vi "controls_disable_status.vi"(8 "Controls[]":refnum<vi>[][](array[refnum]), 11 "motions":T1[](array[typedef])) -> ()   [LabVIEW 2016, in "MotionControl.lvlib"]
uses:
  <userlib>/MotionControl/MotionControl.lvlib
  <userlib>/MotionControl/MotorSystem/MotionCluster.ctl
  <userlib>/MotionControl/OneMotion/OneMotion.lvclass
  <userlib>/MotionControl/MotorSystem/MotorSystem.lvclass
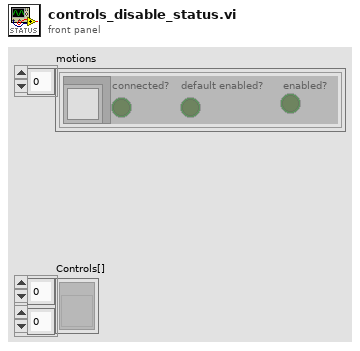
[diagram p1: front panel]
types:
  T1 = typedef "MotionControl.lvlib/MotorSystem.lvclass/MotionCluster.ctl" = cluster{"OneMotion.lvclass":refnum<class "OneMotion.lvclass">, "connected?":bool, "default enabled?":bool, "enabled?":bool}
  T2 = enum8{"Enabled", "Disabled", "Disabled and Grayed Out"}
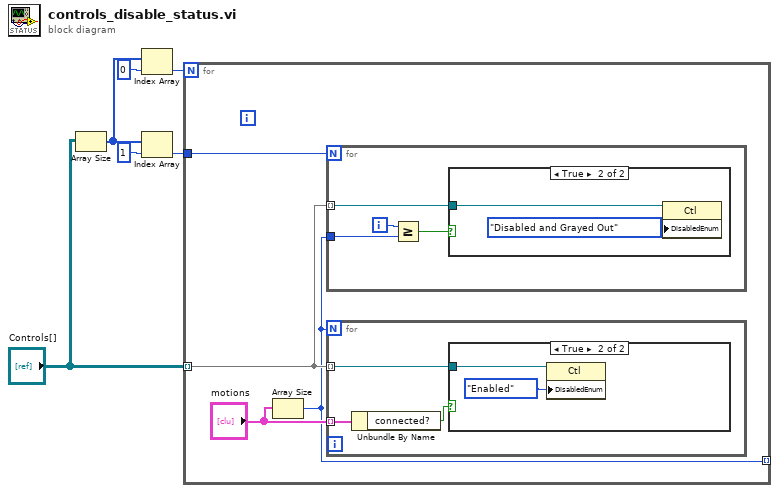
[diagram p0: block diagram]
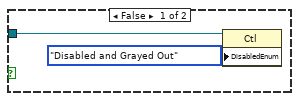
[diagram p3: hidden frame]
diagram:
  n1 = Array Size(array="Controls[]") -> (size(s)=w2:i32[])
  n2 = Index Array(array=w2, index=0 ("索引")) -> (element=w4:i32)
  n3 = Index Array(array=w2, index=1 ("索引")) -> (element=w1:i32)
  n4 = for {
    N: w4 -> [_]
    tunnel: "Controls[]" -> [w10] mode=indexing
    tunnel: [w7] -> _ mode=indexing
    tunnel: w1 -> [w9]
    n5 = Array Size(array="motions") -> (size(s)=w7:i32)
    n6 = for {
      N: w9 -> [_]
      tunnel: w10 -> [w14] mode=indexing
      tunnel: w7 -> [w12]
      i -> [w13]
      n7 = Greater Or Equal?(x=w13, y=w12) -> (x >= y?=w11:bool)
      n8 = case shown="True" w11 {
        tunnel: w14 -> [_ w15]
        frame False {
        }
        frame True {
          n9 = property class="Ctl"(reference=w15, "DisabledEnum"=T2."Disabled and Grayed Out" ("禁用")) -> ()  [unwired: 1 in, 2 out]
        }
      }
    }
    n10 = for {
      N: w7 -> [_]
      tunnel: w10 -> [w18] mode=indexing
      tunnel: "motions" -> [w17] mode=indexing
      n11 = Unbundle By Name(w17) -> ("connected?"=w19:bool)
      n12 = case shown="True" w19 {
        tunnel: w18 -> [w20 w22]
        frame False {
          n13 = property class="Ctl"(reference=w20, "DisabledEnum"=T2."Disabled and Grayed Out" ("禁用")) -> ()  [unwired: 1 in, 2 out]
        }
        frame True {
          n14 = property class="Ctl"(reference=w22, "DisabledEnum"=T2."Enabled" ("禁用")) -> ()  [unwired: 1 in, 2 out]
        }
      }
    }
  }
